vi "UpLoadTempSensorParam332.vi"(5 "Input":u8(ring) caption="Entrées" items=["A", "B"], 6 "Error in":errorcluster, 7 "SensorParIn":T1={"TableTC"=1, "TableConv"=1, "Compensation"=1, "Type"=9} caption="Paramètre de configuration d'entrée In" {"Compensation" items=["Off", "On"]; "TableConv" max=60 step=1; "Type" items=["Silicon Diode", "GaAlAs Diode", "Platinum 100 (250 Ohms)", "Platinum 100 (500 Ohms)", "Platinum 1000 Ohms", "NTC RTD 75mV 7.5 KOhms", "Thermocouple 25mV", "Thermocouple 50mV", "NTC RTD 75mV 75 Ohms", "NTC RTD 75mV 750 Ohms", "NTC RTD 75mV 7.5 KOhms", "NTC RTD 75mV 75 KOhms", "NTC RTD 75mV Auto"]; "TableTC" max=41 step=1}, 9 "VISA Rsrc":refnum<visa-resource-name>="GPIB0::12::INSTR" caption="Nom de la ressource VISA") -> (1 "Error out":errorcluster, 3 "Commnad String":string)   [LabVIEW 2012]
doc: "Ce VI charge les paramêtres de configuration sélectionnées dans le contrôlleur pour l'entrée spécifiée"
uses:
  <userlib>/LSCI 332 V2/InConfigPar332.ctl
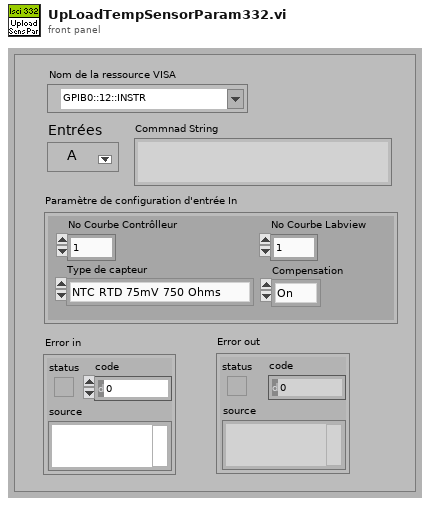
[diagram p1: front panel]
types:
  T1 = typedef "InConfigPar332.ctl" = cluster{"TableTC":u16, "TableConv":u16, "Compensation":u16, "Type":u16}
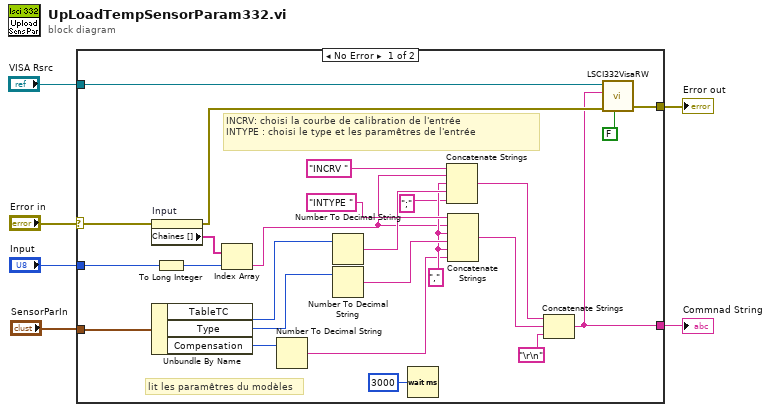
[diagram p0: block diagram]
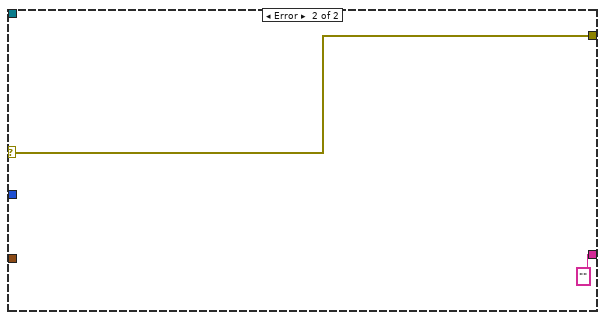
[diagram p2: hidden frame]
diagram:
  n1 = case shown="No Error" "Error in" {
    selector: "Error in" -> [w18 w33]
    tunnel: "VISA Rsrc" -> [w13 _]
    tunnel: "Input" -> [w30 _]
    tunnel: "SensorParIn" -> [w17 _]
    tunnel: [w7 ""] -> w4
    tunnel: [w14 w33] -> w3
    frame No Error {
      w22 = ","
      # "lit les paramêtres du modèles"
      # "INCRV: choisi la courbe de calibration de l'entrée\nINTYPE : choisi le type et les paramêtres de l'entrée"
      n2 = property on="Input" class="Ring (strict)"(error in=w18) -> (error out=w15:errorcluster, "Chaînes []"=w31:string[])  [unwired: 1 in, 1 out]
      n3 = Unbundle By Name(w17) -> ("TableTC"=w27:u16, "Type"=w26:u16, "Compensation"=w20:u16)
      n4 = To Long Integer(number=w30) -> (32bit integer=w29:i32)
      n5 = Index Array(array=w31, index=w29) -> (element=w21:string)
      n6 = Number To Decimal String(number=w20) -> (decimal integer string=w11:string)  [unwired: 1 in]
      n7 = Number To Decimal String(number=w27) -> (decimal integer string=w24:string)  [unwired: 1 in]
      n8 = Number To Decimal String(number=w26) -> (decimal integer string=w23:string)  [unwired: 1 in]
      n9 = Wait (ms)(milliseconds to wait=u32 3000) -> ()  [unwired: 1 out]
      n10 = Concatenate Strings("INCRV ", w21, w22, w24, ";" ("string")) -> (w10:string)
      n11 = Concatenate Strings("INTYPE ", w21, w22, w23, w22, w11) -> (w9:string)
      n12 = Concatenate Strings(w10, w9, "\r\n") -> (w7:string)
      n13 = call <userlib>:"LSCI332VisaRW.vi"("Lecture?(T)"=FALSE, "error in (no error)"=w15, "ChaineCom"=w7, "VISA Rsrc"=w13) -> ("error out"=w14:errorcluster)  [unwired: 3 in, 3 out]
    }
    frame Error {
    }
  }
  "Error out" <- w3
  "Commnad String" <- w4
